vi "Event Handle Loop.vi"(8 "error in (no error)":errorcluster, 10 "Stop User Event":refnum<user-event>, 11 "Scenarios Class in":refnum<class "Scenarios Class.lvclass">) -> (0 "error out":errorcluster, 3 "Scenarios Class out":refnum<class "Scenarios Class.lvclass">)   [LabVIEW 2020, in "SECS Scenarios.lvlib" / "Scenarios Class.lvclass"]
uses:
  Scenarios Class.lvclass
  Scenarios Class.lvclass/Scenarios Class.ctl
  SECS Communication/HSMS Class/HSMS Class.lvclass/HSMS Class.ctl
  07-Event Report From Equipment/07-Event Report From Equipment.lvclass
  D:/Dropbox/SECS/SECS_GEM v1.1.0/Com/SECS Scenarios/Scenarios Class/Scenarios Class.lvclass
  07-Event Report From Equipment/07-Event Report From Equipment.lvclass/07-Event Report From Equipment.ctl
  11-Alarm Management/11-Alarm Management.lvclass
  11-Alarm Management/11-Alarm Management.lvclass/11-Alarm Management.ctl
  14-Process Program Creating Editing or Deleting/14-Process Program Creating Editing or Deleting.lvclass
  14-Process Program Creating Editing or Deleting/14-Process Program Creating Editing or Deleting.lvclass/14-Process Program Creating Editing or Deleting.ctl
  21-Material Movement/21-Material Movement.lvclass
  21-Material Movement/21-Material Movement.lvclass/21-Material Movement.ctl
  23-Equipment Sends Information to Host/23-Equipment Sends Information to Host.lvclass
  23-Equipment Sends Information to Host/23-Equipment Sends Information to Host.lvclass/23-Equipment Sends Information to Host.ctl
  24-Host Accepts On-Line Request from Equipment/24-Host Accepts On-Line Request from Equipment.lvclass
  24-Host Accepts On-Line Request from Equipment/24-Host Accepts On-Line Request from Equipment.lvclass/24-Host Accepts On-Line Request from Equipment.ctl
  25-Host Accepts Off-Line/25-Host Accepts Off-Line.lvclass
  25-Host Accepts Off-Line/25-Host Accepts Off-Line.lvclass/25-Host Accepts Off-Line.ctl
  29-Equipment Requests Time Value from Host/29-Equipment Requests Time Value from Host.lvclass
  29-Equipment Requests Time Value from Host/29-Equipment Requests Time Value from Host.lvclass/29-Equipment Requests Time Value from Host.ctl
  33-Update Trace Data/33-Update Trace Data.lvclass
  33-Update Trace Data/33-Update Trace Data.lvclass/33-Update Trace Data.ctl
  07-Event Report From Equipment/Write CEID.vi
  11-Alarm Management/Write ALID.vi
  14-Process Program Creating Editing or Deleting/Write Process Program CEID.vi
  21-Material Movement/Write Material Movement CEID.vi
  23-Equipment Sends Information to Host/Write TID.vi
  23-Equipment Sends Information to Host/Write TEXT.vi
  24-Host Accepts On-Line Request from Equipment/Write Reply Notifier.vi
  25-Host Accepts Off-Line/Write Off-Line.vi
  29-Equipment Requests Time Value from Host/Write Reply Notifier.vi
  33-Update Trace Data/Write S6F1.vi
  33-Update Trace Data/Write Over.vi
  Read HSMS Class.vi
  SECS Communication/HSMS Class/Read Recive User Event.vi
  SECS Communication/HSMS Class/HSMS Class.lvclass
  SECS Communication/SECS-II Class/SECS-II Class.lvclass
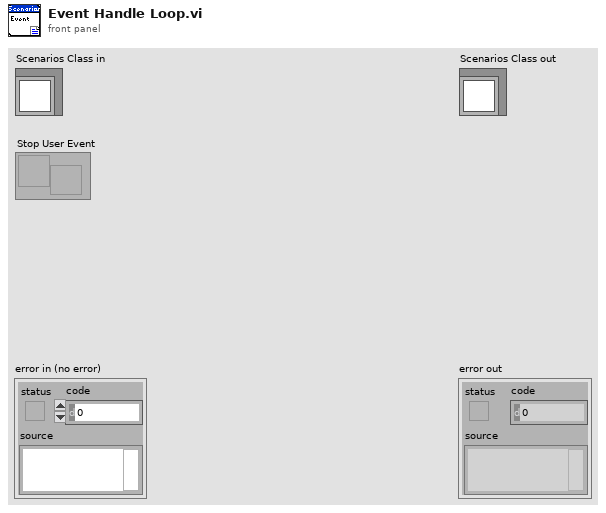
[diagram p1: front panel]
types:
  T1 = typedef "SECS Scenarios.lvlib/Scenarios Class.lvclass/Request Refnum.ctl" = cluster{"11-Alarm Management":refnum<user-event>, "07-Event Report From Equipment":refnum<user-event>, "14-Process Program Creating Editing or Deleting":refnum<user-event>, "21-Material Movement":refnum<user-event>, "23-Equipment Sends Information to Host":refnum<user-event>, "24-Host Accepts On-Line Request from Equipment":refnum<user-event>, "25-Host Refuses On-Line Request":refnum<user-event>, "29-Equipment Requests Time Value from Host":refnum<user-event>, "33-Update Trace Data":refnum<user-event>}
  T2 = typedef "SECS Communication.lvlib/S6 Message Class.lvclass/S6F1.ctl" = cluster{"TRID":u32, "SMPLN":u32, "STIME":string, "SV":cluster{"Format Code":T3, "Value":variant}[]}
  T3 = typedef "SECS Communication.lvlib/SECS-II Class.lvclass/Format Code.ctl" = enum16{"L", "A", "B", "Boolean", "J", "I1", "I2", "I4", "I8", "U1", "U2", "U4", "U8", "F4", "F8", "Char"}
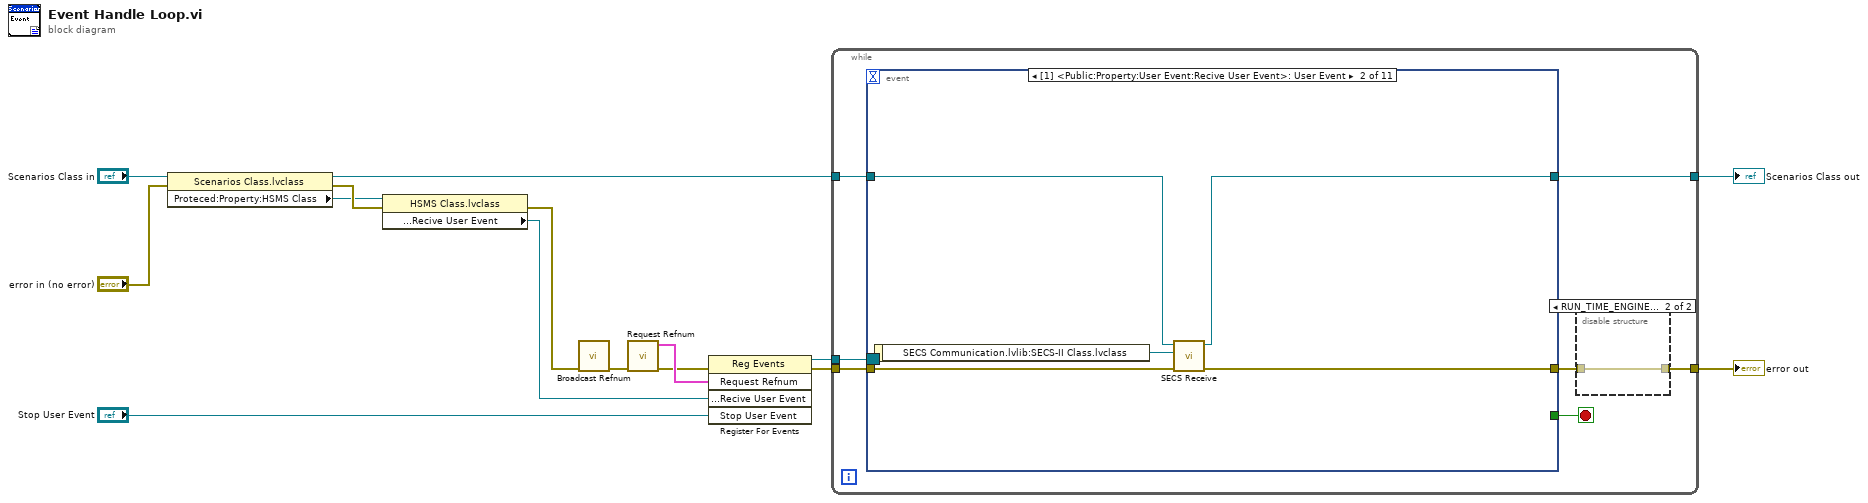
[diagram p0: block diagram]
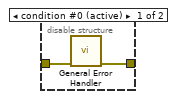
[diagram p2: hidden frame]
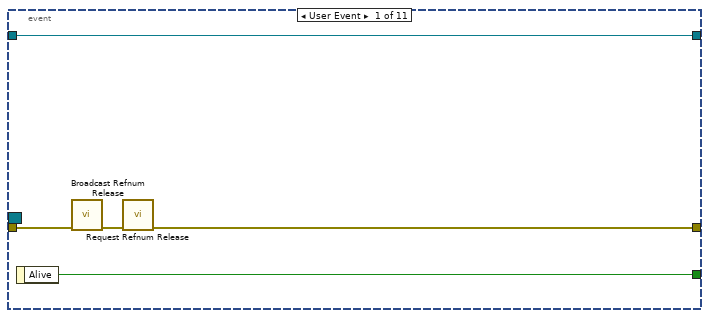
[diagram p3: hidden frame]
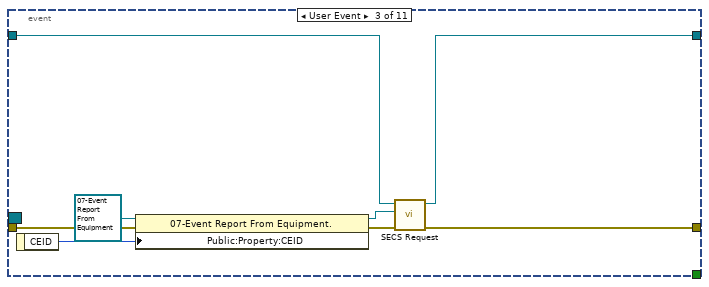
[diagram p4: hidden frame]
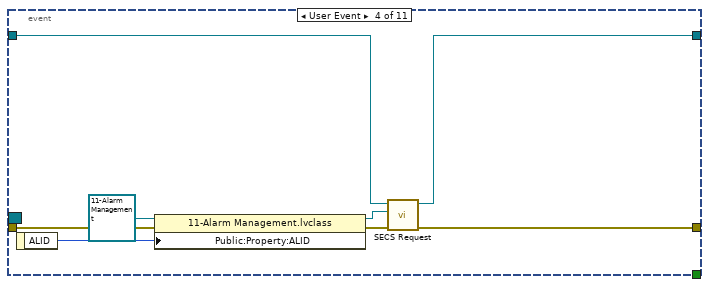
[diagram p5: hidden frame]
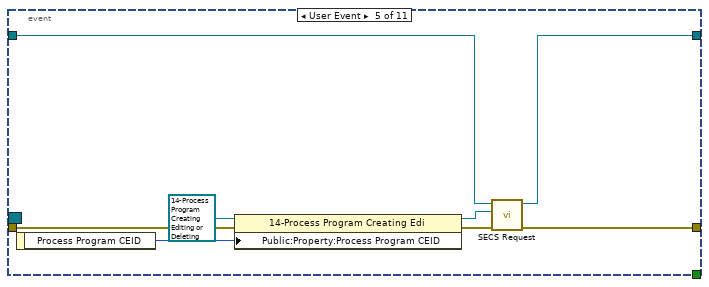
[diagram p6: hidden frame]
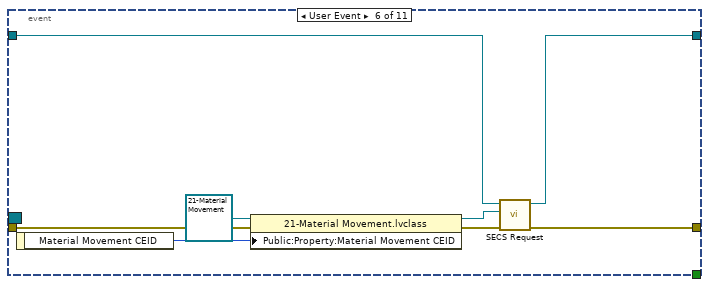
[diagram p7: hidden frame]
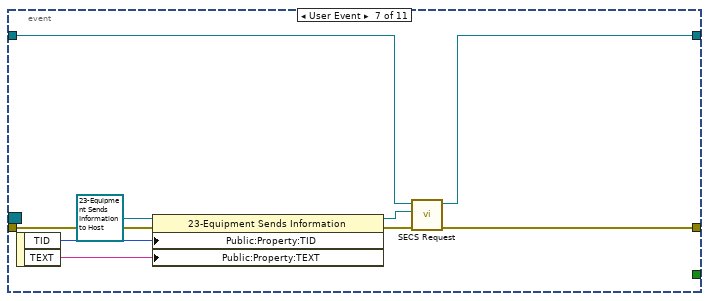
[diagram p8: hidden frame]
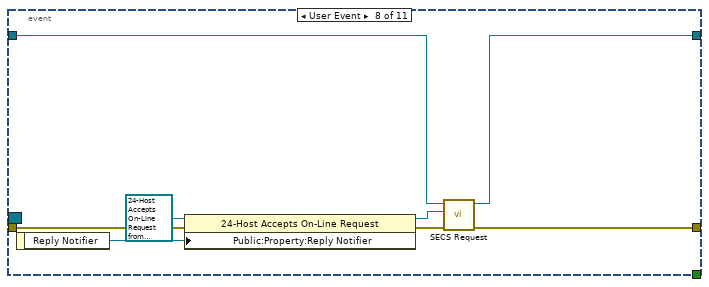
[diagram p9: hidden frame]
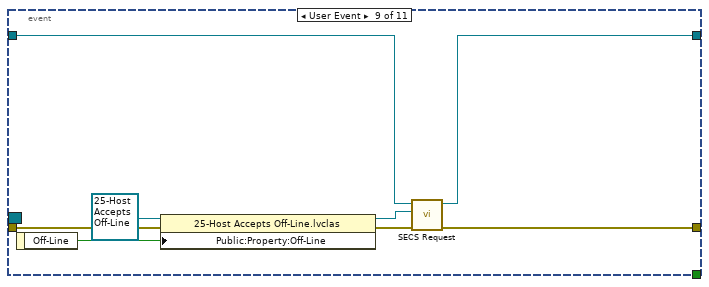
[diagram p10: hidden frame]
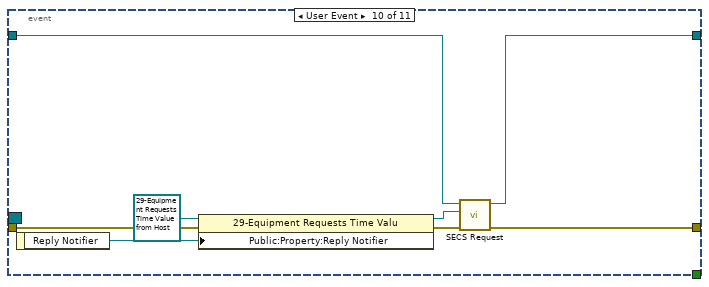
[diagram p11: hidden frame]
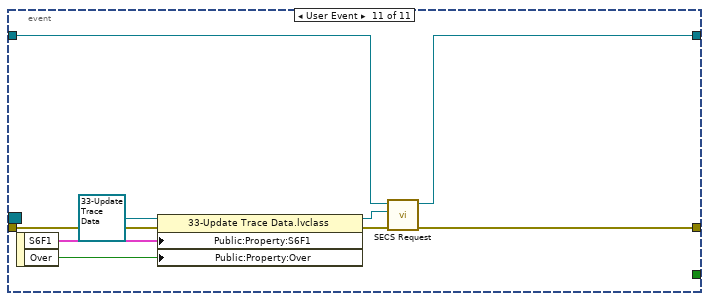
[diagram p12: hidden frame]
diagram:
  n1 = property class="Scenarios Class.lvclass"(reference="Scenarios Class in", error in="error in (no error)") -> (reference out=w7:refnum<class "Scenarios Class.lvclass">, error out=w11:errorcluster, "Proteced:Property:HSMS Class"=w10:refnum<class "HSMS Class.lvclass">)
  n2 = property class="HSMS Class.lvclass"(reference=w10, error in=w11) -> (error out=w9:errorcluster, "Public:Property:User Event:Recive User Event"=w2:refnum<user-event>)  [unwired: 1 out]
  n3 = call "Broadcast Refnum.vi"("error in"=w9) -> ("error out"=w8:errorcluster)  [unwired: 9 in, 1 out]
  n4 = call "Request Refnum.vi"("error in"=w8) -> ("error out"=w4:errorcluster, "Request Refnum"=w13:T1)  [unwired: 9 in]
  n5 = register-events(error in=w4, w13, w2, "Stop User Event") -> (reference out=w5:refnum<event-registration>, error out=w6:errorcluster)  [unwired: 1 in]
  n6 = while {
    tunnel: w6 -> [w22]
    tunnel: w7 -> [w21]
    tunnel: [w20] -> w15
    tunnel: [w16] -> w3
    tunnel: w5 -> [w18]
    stop <- w19 stop-if-true
    n7 = event shown="[1] <Public:Property:User Event:Recive User Event>: User Event" {
      selector: w18 -> [_ _ _ _ _ _ _ _ _ _ _]
      dyn-events: _ -> [_ _ _ _ _ _ _ _ _ _ _]
      timeout: _ -> [_ _ _ _ _ _ _ _ _ _ _]
      tunnel: w22 -> [w28 w35 w43 w51 w59 w67 w76 w84 w92 w100 w109]
      tunnel: w21 -> [w30 w33 w39 w46 w55 w63 w72 w80 w88 w96 w105]
      tunnel: [w30 w32 w36 w45 w54 w62 w71 w79 w87 w95 w104] -> w20
      tunnel: [w26 w31 w37 w44 w53 w61 w70 w78 w86 w94 w103] -> w17
      tunnel: [w29 _ _ _ _ _ _ _ _ _ _] -> w19
      event User Event {
        n8 = event-data() -> ("Alive"=w29:bool)  [unwired: 1 in]
        n9 = call "Broadcast Refnum Release.vi"("error in"=w28) -> ("error out"=w27:errorcluster)  [unwired: 10 in]
        n10 = call "Request Refnum Release.vi"("error in"=w27) -> ("error out"=w26:errorcluster)  [unwired: 10 in]
      }
      event User Event {
        n11 = event-data() -> ("SECS Communication.lvlib:SECS-II Class.lvclass"=w34:refnum<class "SECS-II Class.lvclass">)  [unwired: 1 in]
        n12 = call "SECS Receive.vi"("error in (no error)"=w35, "SECS-II Class"=w34, "Scenarios Class in"=w33) -> ("error out"=w31:errorcluster, "Scenarios Class out"=w32:refnum<class "Scenarios Class.lvclass">)  [unwired: 7 in]
      }
      event User Event {
        n13 = event-data() -> ("CEID"=w41:u32)  [unwired: 1 in]
        n14 = property class="07-Event Report From Equipment."(reference=refnum<class "07-Event Report From Equipment.lvclass"> refnum ("SECS Scenarios.lvlib:07-Event Report From Equipment.lvclass"), error in=w43, "Public:Property:CEID"=w41) -> (reference out=w38:refnum<class "07-Event Report From Equipment.lvclass">, error out=w40:errorcluster)
        n15 = call "SECS Request.vi"("error in (no error)"=w40, "Scenarios Class"=w38, "Scenarios Class in"=w39) -> ("error out"=w37:errorcluster, "Scenarios Class out"=w36:refnum<class "Scenarios Class.lvclass">)  [unwired: 7 in]
      }
      event User Event {
        n16 = event-data() -> ("ALID"=w50:u32)  [unwired: 1 in]
        n17 = property class="11-Alarm Management.lvclass"(reference=refnum<class "11-Alarm Management.lvclass"> refnum ("SECS Scenarios.lvlib:11-Alarm Management.lvclass"), error in=w51, "Public:Property:ALID"=w50) -> (reference out=w47:refnum<class "11-Alarm Management.lvclass">, error out=w48:errorcluster)
        n18 = call "SECS Request.vi"("error in (no error)"=w48, "Scenarios Class"=w47, "Scenarios Class in"=w46) -> ("error out"=w44:errorcluster, "Scenarios Class out"=w45:refnum<class "Scenarios Class.lvclass">)  [unwired: 7 in]
      }
      event User Event {
        n19 = event-data() -> ("Process Program CEID"=w58:u32)  [unwired: 1 in]
        n20 = property class="14-Process Program Creating Edi"(reference=refnum<class "14-Process Program Creating Editing or Deleting.lvclass"> refnum ("SECS Scenarios.lvlib:14-Process Program Creating Editing or Deleting.lvclass"), error in=w59, "Public:Property:Process Program CEID"=w58) -> (reference out=w56:refnum<class "14-Process Program Creating Editing or Deleting.lvclass">, error out=w57:errorcluster)
        n21 = call "SECS Request.vi"("error in (no error)"=w57, "Scenarios Class"=w56, "Scenarios Class in"=w55) -> ("error out"=w53:errorcluster, "Scenarios Class out"=w54:refnum<class "Scenarios Class.lvclass">)  [unwired: 7 in]
      }
      event User Event {
        n22 = event-data() -> ("Material Movement CEID"=w66:u32)  [unwired: 1 in]
        n23 = property class="21-Material Movement.lvclass"(reference=refnum<class "21-Material Movement.lvclass"> refnum ("SECS Scenarios.lvlib:21-Material Movement.lvclass"), error in=w67, "Public:Property:Material Movement CEID"=w66) -> (reference out=w64:refnum<class "21-Material Movement.lvclass">, error out=w65:errorcluster)
        n24 = call "SECS Request.vi"("error in (no error)"=w65, "Scenarios Class"=w64, "Scenarios Class in"=w63) -> ("error out"=w61:errorcluster, "Scenarios Class out"=w62:refnum<class "Scenarios Class.lvclass">)  [unwired: 7 in]
      }
      event User Event {
        n25 = event-data() -> ("TID"=w75:u8, "TEXT"=w68:string)  [unwired: 1 in]
        n26 = property class="23-Equipment Sends Information "(reference=refnum<class "23-Equipment Sends Information to Host.lvclass"> refnum ("SECS Scenarios.lvlib:23-Equipment Sends Information to Host.lvclass"), error in=w76, "Public:Property:TID"=w75, "Public:Property:TEXT"=w68) -> (reference out=w73:refnum<class "23-Equipment Sends Information to Host.lvclass">, error out=w74:errorcluster)
        n27 = call "SECS Request.vi"("error in (no error)"=w74, "Scenarios Class"=w73, "Scenarios Class in"=w72) -> ("error out"=w70:errorcluster, "Scenarios Class out"=w71:refnum<class "Scenarios Class.lvclass">)  [unwired: 7 in]
      }
      event User Event {
        n28 = event-data() -> ("Reply Notifier"=w83:refnum<notifier>)  [unwired: 1 in]
        n29 = property class="24-Host Accepts On-Line Request"(reference=refnum<class "24-Host Accepts On-Line Request from Equipment.lvclass"> refnum ("SECS Scenarios.lvlib:24-Host Accepts On-Line Request from Equipment.lvclass"), error in=w84, "Public:Property:Reply Notifier"=w83) -> (reference out=w81:refnum<class "24-Host Accepts On-Line Request from Equipment.lvclass">, error out=w82:errorcluster)
        n30 = call "SECS Request.vi"("error in (no error)"=w82, "Scenarios Class"=w81, "Scenarios Class in"=w80) -> ("error out"=w78:errorcluster, "Scenarios Class out"=w79:refnum<class "Scenarios Class.lvclass">)  [unwired: 7 in]
      }
      event User Event {
        n31 = event-data() -> ("Off-Line"=w91:bool)  [unwired: 1 in]
        n32 = property class="25-Host Accepts Off-Line.lvclas"(reference=refnum<class "25-Host Accepts Off-Line.lvclass"> refnum ("SECS Scenarios.lvlib:25-Host Refuses On-Line Request.lvclass"), error in=w92, "Public:Property:Off-Line"=w91) -> (reference out=w89:refnum<class "25-Host Accepts Off-Line.lvclass">, error out=w90:errorcluster)
        n33 = call "SECS Request.vi"("error in (no error)"=w90, "Scenarios Class"=w89, "Scenarios Class in"=w88) -> ("error out"=w86:errorcluster, "Scenarios Class out"=w87:refnum<class "Scenarios Class.lvclass">)  [unwired: 7 in]
      }
      event User Event {
        n34 = event-data() -> ("Reply Notifier"=w99:refnum<notifier>)  [unwired: 1 in]
        n35 = property class="29-Equipment Requests Time Valu"(reference=refnum<class "29-Equipment Requests Time Value from Host.lvclass"> refnum ("SECS Scenarios.lvlib:29-Equipment Requests Time Value from Host.lvclass"), error in=w100, "Public:Property:Reply Notifier"=w99) -> (reference out=w97:refnum<class "29-Equipment Requests Time Value from Host.lvclass">, error out=w98:errorcluster)
        n36 = call "SECS Request.vi"("error in (no error)"=w98, "Scenarios Class"=w97, "Scenarios Class in"=w96) -> ("error out"=w94:errorcluster, "Scenarios Class out"=w95:refnum<class "Scenarios Class.lvclass">)  [unwired: 7 in]
      }
      event User Event {
        n37 = event-data() -> ("S6F1"=w108:T2, "Over"=w101:bool)  [unwired: 1 in]
        n38 = property class="33-Update Trace Data.lvclass"(reference=refnum<class "33-Update Trace Data.lvclass"> refnum ("SECS Scenarios.lvlib:33-Update Trace Data.lvclass"), error in=w109, "Public:Property:S6F1"=w108, "Public:Property:Over"=w101) -> (reference out=w106:refnum<class "33-Update Trace Data.lvclass">, error out=w107:errorcluster)
        n39 = call "SECS Request.vi"("error in (no error)"=w107, "Scenarios Class"=w106, "Scenarios Class in"=w105) -> ("error out"=w103:errorcluster, "Scenarios Class out"=w104:refnum<class "Scenarios Class.lvclass">)  [unwired: 7 in]
      }
    }
    n40 = disable-structure shown="RUN_TIME_ENGINE==True" {
      disable-tunnel: w17 -> [w24 w25]
      disable-tunnel: [w23 w25] -> w16
      frame condition #0 (active) {
        n41 = call <vilib>:"General Error Handler.vi"("error in (no error)"=w24) -> ("error out"=w23:errorcluster)  [unwired: 10 in, 4 out]
      }
      frame condition #1 {
      }
    }
  }
  "error out" <- w3
  "Scenarios Class out" <- w15
